vi "Ic_Zernike.vi"(5 "Coeff":dbl, 6 "Pixel Pitch 0:20um_or_ 1:12.5um":i32, 7 "diameter / mm":dbl, 8 "error in (no error)":errorcluster, 9 "n":i32, 10 "m":i32, 11 "2D array in (LCOS size buf)":u8[][](array[numeric])) -> (0 "error out":errorcluster, 3 "2D array out":u8[][](array[numeric]))   [LabVIEW 2016]
uses:
  SLM_Control_VI_source/Image_Control.dll
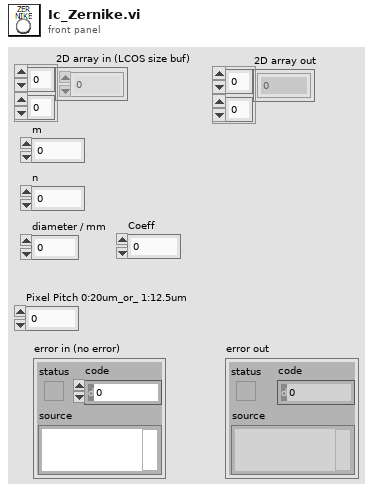
[diagram p1: front panel]
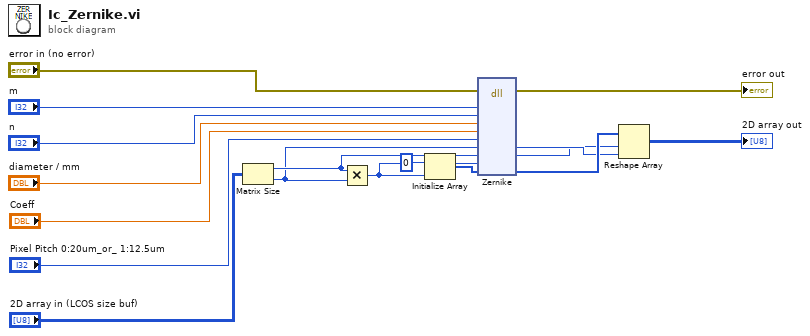
[diagram p0: block diagram]
diagram:
  n1 = Matrix Size(0:"2D array in (LCOS size buf)") -> (1:w4:i32, 2:w3:i32)
  n2 = Multiply(x=w4, y=w3) -> (x*y=w10:i32)
  n3 = Initialize Array(u8 0 ("要素"), w10) -> (w9:u8[])
  n4 = dll-call lib="C:/Users/hs5921/Desktop/SLM_Control_VI_source/Image_Control.dll" fn="Zernike"(error in="error in (no error)", "m"="m", "n"="n", "diameter / mm"="diameter / mm", "Coeff"="Coeff", "PixelPitch0:20um_or_1:12.5um"="Pixel Pitch 0:20um_or_ 1:12.5um", "X_pixel_target"=w3, "Y_pixel_target"=w4, "targetDataSize"=w10, "1DArrayOut"=w9) -> (error out=→"error out":errorcluster, "X_pixel_target"=w7:i32, "Y_pixel_target"=w6:i32, "1DArrayOut"=w8:u8[])  [unwired: 9 in, 1 out]
  n5 = Reshape Array(w8, w6, w7) -> (→"2D array out":u8[][])
